vi "DMM_Close Reference.vi"(8 "error in (no error)":errorcluster, 11 "User Reference":T1) -> (0 "error out":errorcluster)   [LabVIEW 2018, in "DMM Virtual.lvclass"]
uses:
  DMM Virtual.lvclass
  Controls/User Reference.ctl
  DMM_Global.vi
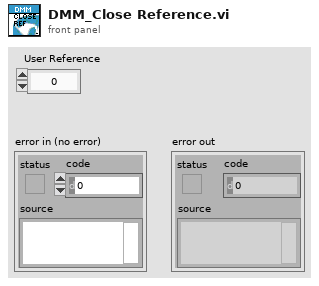
[diagram p1: front panel]
types:
  T1 = typedef "User Reference.ctl" = i32
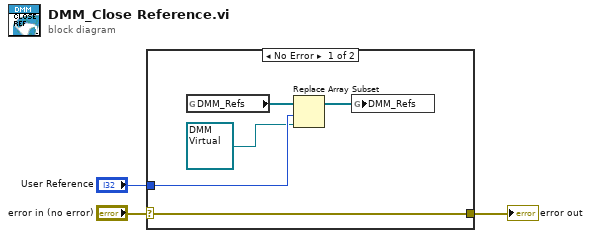
[diagram p0: block diagram]
diagram:
  n1 = case shown="No Error" "error in (no error)" {
    selector: "error in (no error)" -> [w8 w9]
    tunnel: [w8 w9] -> w2
    tunnel: "User Reference" -> [w6 _]
    frame No Error {
      n2 = global read "DMM_Global.vi" "DMM_Refs"() -> (w7:refnum<class "DMM Virtual.lvclass">[])
      n3 = Replace Array Subset(array=w7, new element=refnum<class "DMM Virtual.lvclass"> refnum ("DMM Virtual.lvclass"), index=w6) -> (w5:refnum<class "DMM Virtual.lvclass">[])
      n4 = global write "DMM_Global.vi" "DMM_Refs"(w5) -> ()
    }
    frame Error {
    }
  }
  "error out" <- w2
